vi "Exercises_5-1-3.vi"() -> ()   [LabVIEW 2014]
panel:
  out "Second Column":dbl[](array[numeric])
  out "Third Row":dbl[](array[numeric])
  out "Array":dbl[][](array[numeric])
  in  "Colums":i32
  in  "Rows":i32
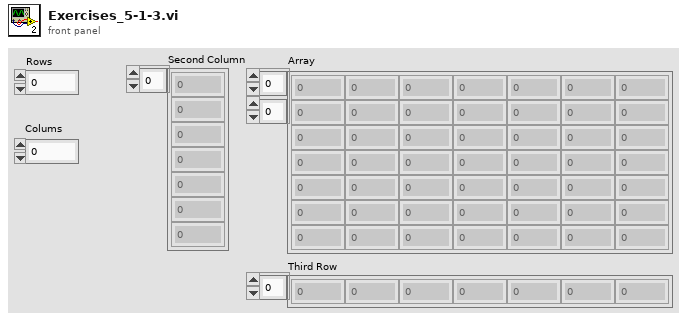
[diagram p1: front panel]
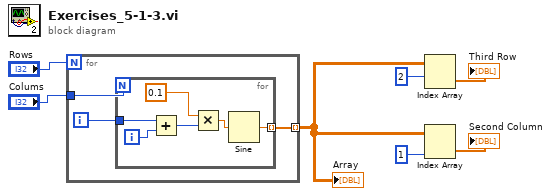
[diagram p0: block diagram]
diagram:
  n1 = for {
    N: "Rows" -> [_]
    tunnel: "Colums" -> [w10]
    tunnel: [w8] -> w5 mode=indexing
    i -> [w9]
    n2 = for {
      N: w10 -> [_]
      tunnel: w9 -> [w16]
      tunnel: [w11] -> w8 mode=indexing
      i -> [w15]
      n3 = Add(x=w16, y=w15) -> (x+y=w13:i32)
      n4 = Multiply(x=0.1, y=w13) -> (x*y=w12:dbl)
      n5 = Sine(x=w12) -> (sin(x)=w11:dbl)
    }
  }
  "Array" <- w5
  n6 = Index Array(array=w5, index (row)=2) -> (element=→"Third Row":dbl[])  [unwired: 1 in]
  n7 = Index Array(array=w5, index (col)=1) -> (element=→"Second Column":dbl[])  [unwired: 1 in]
